vi "ArrayToEnum.vi"(7 "Control VI Type (control)":T1=enum."control" caption="Control VI Type", 8 "Error In":errorcluster, 9 "Enum Name (Enum)":string caption="Enum Name (FileName)", 10 "Enum Strings":string[](array[string]), 11 "Control Path":path caption="Control Path (use dialog)") -> (0 "Error Out":errorcluster)   [LabVIEW 2021, in "Update Enum.lvlib"]
doc: "This VI converts an array of strings into an enum with the strings as enum value-strings\n\nVariant to Control\nCopyright © 2007, Ton Plomp\nAll rights reserved.\ntcplomp@gmail.com\n\nDistribution:\nThis code was downloaded from:\nhttp://forums.lavag.org/downloads-file89.html\n\nDescription::\nOriginated from Array To Enum\n\nAcknowledgements:\nUses code by Bob Billier from his RTM to Enum tool (http://forums.lavag.org/downloads-file72.html)\n\nDependencies:\nUses the following OpenG toolkits:\noglib_lvdata-2.7-1\noglib_error-2.3-1\noglib_file-2.8-1\n\nThese can be installed with VIPM (http://jkisoft.com/VIPM)\n\nLicense:\nDistributed under the BSD license."
uses:
  Update Enum.lvlib
  typdef/ControlTypes.ctl
  <userlib>/_OpenG.lib/lvdata/lvdata.llb/openg_variant.lvlib
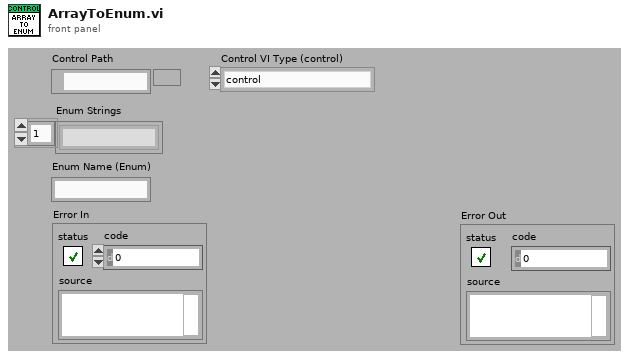
[diagram p1: front panel]
types:
  T1 = typedef "Update Enum.lvlib/ControlTypes.ctl" = enum32{"not a control VI", "control", "typedef", "strict typedef"}
  T2 = enum32{"invalid VI type", "Standard VI", "Control VI", "Global VI", "Polymorphic VI"}
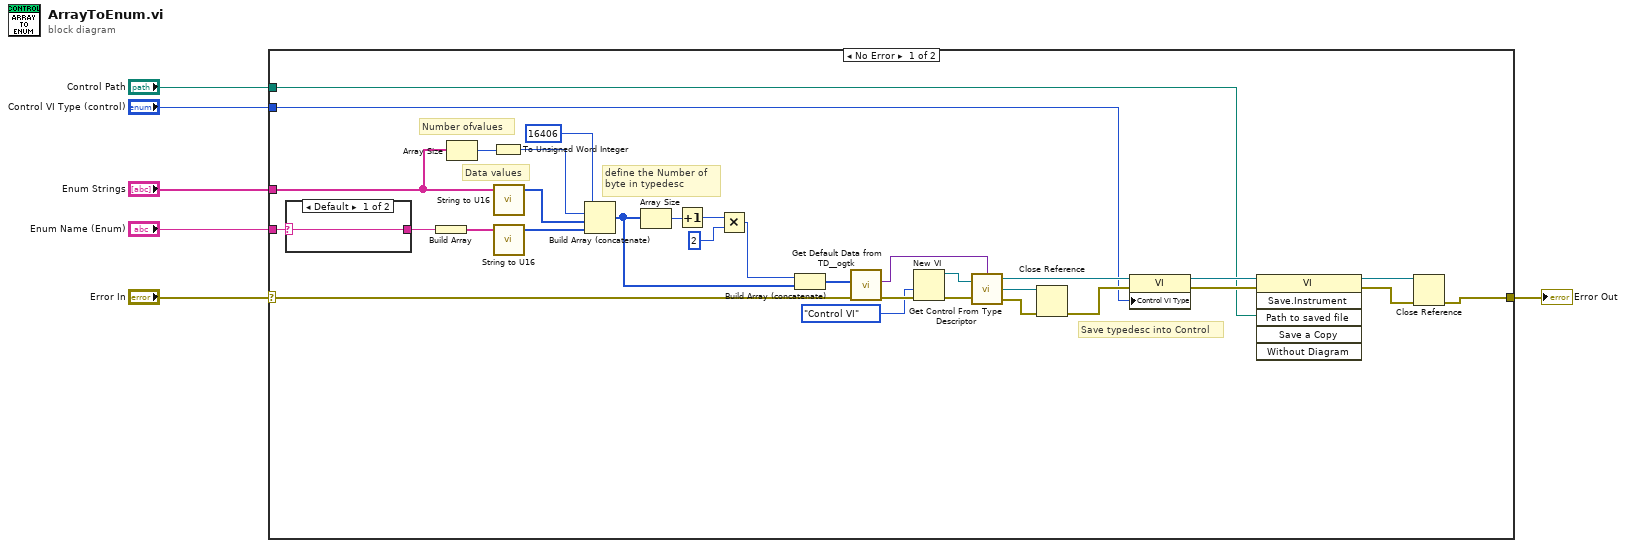
[diagram p0: block diagram]
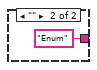
[diagram p2: hidden frame]
diagram:
  n1 = case shown="No Error" "Error In" {
    selector: "Error In" -> [w27 w41]
    tunnel: "Enum Strings" -> [w26 _]
    tunnel: "Enum Name (Enum)" -> [w38 _]
    tunnel: [w12 w41] -> w4
    tunnel: "Control VI Type (control)" -> [w13 _]
    tunnel: "Control Path" -> [w10 _]
    frame No Error {
      # "Save typedesc into Control"
      # "Data values"
      # "Number ofvalues"
      # "define the Number of\nbyte in typedesc"
      n2 = case shown="Default" w38 {
        selector: w38 -> [w39 _]
        tunnel: [w39 "Enum"] -> w29
        frame Default {
        }
        frame "" {
        }
      }
      n3 = Build Array(w29) -> (w24:string[])
      n4 = Array Size(array=w26) -> (size(s)=w31:i32)
      n5 = To Unsigned Word Integer(number=w31) -> (unsigned 16bit integer=w30:u16)
      n6 = call "String to U16.vi"("Array of Strings"=w26) -> ("Array of U16"=w25:u16[])  [unwired: 4 in]
      n7 = call "String to U16.vi"("Array of Strings"=w24) -> ("Array of U16"=w23:u16[])  [unwired: 4 in]
      n8 = Build Array (concatenate)(u16 16406, w30, w25, w23) -> (w33:u16[])
      n9 = Array Size(array=w33) -> (size(s)=w37:i32)
      n10 = Increment(x=w37) -> (x+1=w36:i32)
      n11 = Multiply(x=w36, y=2) -> (x*y=w34:i32)
      n12 = Build Array (concatenate)(w34, w33) -> (w28:i32[])
      n13 = call <userlib>:"Get Default Data from TD__ogtk.vi"("error in (no error)"=w27, "Type Descriptor"=w28) -> ("error out"=w14:errorcluster, "Default VData"=w8:variant)  [unwired: 8 in]
      n14 = New VI(8:w14, 9:T2."Control VI" ("vi type (standard vi)")) -> (0:w22:errorcluster, 3:w9:refnum<vi>)  [unwired: 5 in]
      n15 = call "Get Control From Type Descriptor.vi"("VI Refnum"=w9, "error in (no error)"=w22, "data type"=w8) -> ("VI Refnum"=w15:refnum<vi>, "New Control Ref"=w20:refnum<vi>, "error out"=w19:errorcluster)
      n16 = Close Reference(reference=w20, error in (no error)=w19) -> (error out=w18:errorcluster)
      n17 = property class="VI"(reference=w15, error in=w18, "Control VI Type"=w13) -> (reference out=w16:refnum<vi>, error out=w17:errorcluster)
      n18 = invoke class="VI" method="Save.Instrument"(reference=w16, error in=w17, "Path to saved file"=w10) -> (reference out=w21:refnum<vi>, error out=w11:errorcluster)  [unwired: 3 in, 4 out]
      n19 = Close Reference(reference=w21, error in (no error)=w11) -> (error out=w12:errorcluster)
    }
    frame Error {
    }
  }
  "Error Out" <- w4
